vi "Ch_Active_Control.vi"(2 "Match":string, 3 "Activate Channels?":bool, 4 "Client Name":string="G3_3 HD", 5 "Control on":enum16{"Channel Name", "Main Address"}(ring)) -> (0 "Editted Channels":T1[](array[typedef]) {"Duty" format="%.0b"; "D" format="%#_5g"; "C" format="%#_5g"; "B" format="%#_5g"; "A" format="%#_5g"}, 1 "No of Channels":i32)   [LabVIEW 2013]
uses:
  ADAM Client/Sub VIs/ADAM Controls/Ch_description_ADAM.ctl
  ADAM Client/Sub VIs/ADAM Controls/Module_type_ADAM.ctl
  ADAM Client/Sub VIs/ADAM Controls/Function_ADAM.ctl
  ADAM Client/Sub VIs/ADAM Controls/Channel_State.ctl
  ADAM Client/Sub VIs/ADAM Controls/Calib_type_ADAM.ctl
  ADAM Client/Sub VIs/ADAM Controls/Address.ctl
  Sub VI's/Channel_Description_Global.vi
  Anemometry/Anemometry Sub Vis/Globals/Preference_global.vi
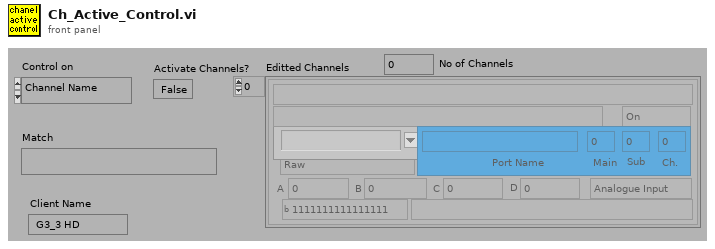
[diagram p1: front panel]
types:
  T1 = typedef "Ch_description_ADAM.ctl" = cluster{"Ch Name":string, "Type":T2, "Function":T3, "Ch State":T4, "Calibration type":T5, "A":dbl, "B":dbl, "C":dbl, "D":dbl, "Comments":string, "Address":T6, "String":string, "Duty":u16}
  T2 = typedef "Module_type_ADAM.ctl" = string
  T3 = typedef "Function_ADAM.ctl" = enum16{"Analogue Input", "Digital Input", "Event counter", "Event rate", "Analogue Output", "Digital Output", "Relay Output"}
  T4 = typedef "Channel_State.ctl" = enum16{"On", "Off", "Always On", "Always Off"}
  T5 = typedef "Calib_type_ADAM.ctl" = enum16{"Raw", "Bx + A", "Cx^2 + Bx + A", "Dx^3 + Cx^2 + Bx + A", "In Band", "Hi-Tec Q", "Hi-Tec M_dot", "Text"}
  T6 = typedef "Address.ctl" = cluster{"Main":i32, "Ch.":i32, "Sub":i32, "Port Name":string}
  T7 = enum16{"Append to Global", "Read Global then Clear"}
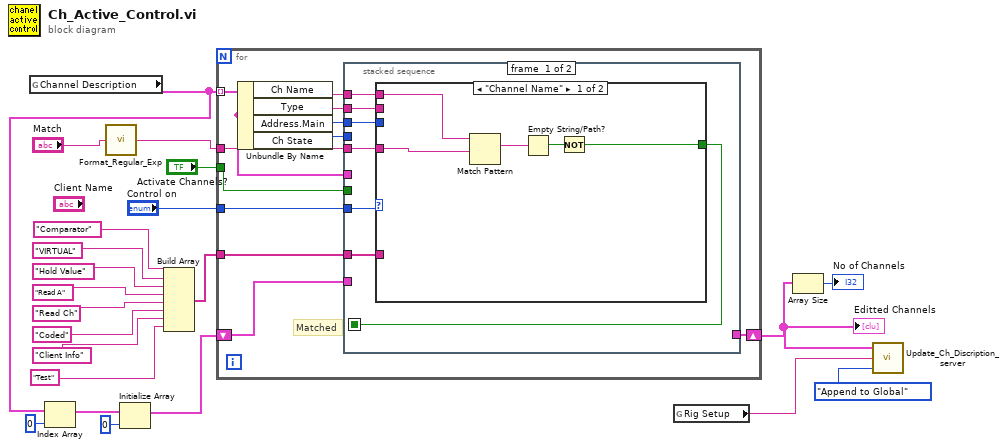
[diagram p0: block diagram]
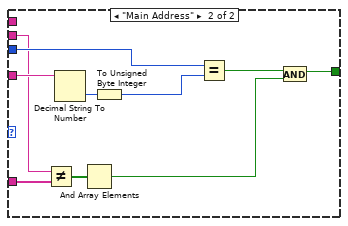
[diagram p2: hidden frame]
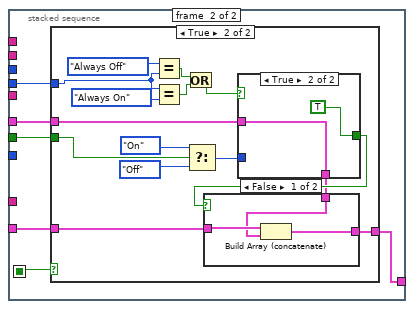
[diagram p3: hidden frame]
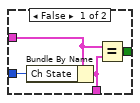
[diagram p6: hidden frame]
diagram:
  n1 = global read "Channel_Description_Global.vi" "Channel Description"() -> (w4:T1[])
  n2 = Index Array(array=w4, index=0 ("Index")) -> (element=w10:T1)
  n3 = call "Format_Regular_Exp.vi"("Regular expression"="Match") -> ("Case Insensitive for html"=w1:string)
  n4 = Initialize Array(w10, 0 ("Dimension Size")) -> (w8:T1[])
  n5 = Build Array(T2 "Comparator" ("Type"), T2 "VIRTUAL" ("Type"), T2 "Hold Value" ("Type"), T2 "Read A" ("Type"), T2 "Read Ch" ("Type"), T2 "Coded" ("Type"), T2 "Client Info" ("Type"), T2 "Test" ("Type")) -> (w13:T2[])
  n6 = for {
    tunnel: w4 -> [w26] mode=indexing
    tunnel: "Control on" -> [w33]
    tunnel: w1 -> [w32]
    tunnel: w13 -> [w28]
    tunnel: "Activate Channels?" -> [w25]
    shift-right: [w23] -> w6
    shift-left: w8 -> [w24]
    # "Matched"
    n7 = Unbundle By Name(w26) -> ("Ch Name"=w31:string, "Type"=w29:T2, "Address.Main"=w30:i32, "Ch State"=w27:T4)
    n8 = stacked-sequence {
      seq-local: [w37 _] -> [_ w61]
      tunnel: w33 -> [w40 _]
      tunnel: w32 -> [w39 _]
      tunnel: w31 -> [w38 _]
      tunnel: w30 -> [w36 _]
      tunnel: w29 -> [w35 _]
      tunnel: w28 -> [w34 _]
      tunnel: w27 -> [_ w60]
      tunnel: w26 -> [_ w59]
      tunnel: w25 -> [_ w58]
      tunnel: w24 -> [_ w57]
      tunnel: [_ w56] -> w23
      frame #0 {
        n9 = case shown="\"Channel Name\"" w40 {
          tunnel: w39 -> [w45 w55]
          tunnel: w38 -> [w44 _]
          tunnel: [w41 w46] -> w37
          tunnel: w36 -> [_ w53]
          tunnel: w35 -> [_ w51]
          tunnel: w34 -> [_ w50]
          frame "Channel Name" {
            n10 = Match Pattern(string=w44, regular expression=w45) -> (match substring=w43:string)  [unwired: 4 out]
            n11 = Empty String/Path?(string/path=w43) -> (empty?=w42:bool)
            n12 = Not(x=w42) -> (.not. x?=w41:bool)
          }
          frame "Main Address" {
            n13 = Not Equal?(x=w51, y=w50) -> (x != y?=w49:bool[])
            n14 = Decimal String To Number(string=w55) -> (number=w54:i32)  [unwired: 3 out]
            n15 = And Array Elements(Boolean array=w49) -> (logical AND=w47:bool)
            n16 = To Unsigned Byte Integer(number=w54) -> (unsigned 8bit integer=w52:u8)
            n17 = Equal?(x=w53, y=w52) -> (x = y?=w48:bool)
            n18 = And(x=w48, y=w47) -> (x .and. y?=w46:bool)
          }
        }
      }
      frame #1 {
        n19 = case shown="True" w61 {
          tunnel: w60 -> [_ w71]
          tunnel: w59 -> [_ w77]
          tunnel: w58 -> [_ w73]
          tunnel: w57 -> [w62 w65]
          tunnel: [w62 w64] -> w56
          frame False {
          }
          frame True {
            n20 = Equal?(x=Channel_State."Always Off" ("Channel State"), y=w71) -> (x = y?=w68:bool)
            n21 = Equal?(x=w71, y=Channel_State."Always On" ("Channel State")) -> (x = y?=w69:bool)
            n22 = Or(x=w68, y=w69) -> (x .or. y?=w67:bool)
            n23 = Select(t=Channel_State."On" ("Channel State"), s=w73, f=Channel_State."Off" ("Channel State")) -> (s? t:f=w74:T4)
            n24 = case shown="True" w67 {
              tunnel: w77 -> [w84 w86]
              tunnel: w74 -> [w85 _]
              tunnel: [w83 TRUE] -> w66
              tunnel: [w82 w86] -> w63
              frame False {
                n25 = Bundle By Name(cluster=w84, "Ch State"=w85) -> (w82:T1)
                n26 = Equal?(x=w84, y=w82) -> (x = y?=w83:bool)
              }
              frame True {
              }
            }
            n27 = case shown="False" w66 {
              tunnel: w65 -> [w80 w81]
              tunnel: [w79 w81] -> w64
              tunnel: w63 -> [w78 _]
              frame False {
                n28 = Build Array (concatenate)(w80, w78) -> (w79:T1[])
              }
              frame True {
              }
            }
          }
        }
      }
    }
  }
  "Editted Channels" <- w6
  n29 = global read "Preference_global.vi" "Rig Setup"() -> (w3:string)
  n30 = Array Size(array=w6) -> (size(s)=→"No of Channels":i32)
  n31 = call "Update_Ch_Discription_server.vi"("Mode"=T7."Append to Global", "Client HD name"=w3, "Channels to update In"=w6) -> ()  [unwired: 1 out]
